vi "MKS_PDR2000_write_read.vi"(0 "PDR2000 COM port":refnum<visa-resource-name>, 2 "Write string":string, 11 "error in (no error)":errorcluster) -> (4 "PDR2000 COM port out":refnum<visa-resource-name>, 13 "Read String":string, 15 "error out":errorcluster)   [LabVIEW 2019]
uses:
  <vilib>/regexp/Match Regular Expression.xnode
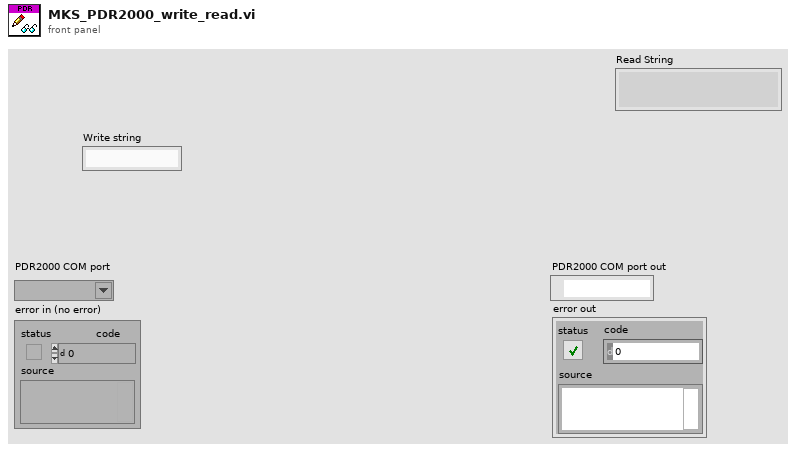
[diagram p1: front panel]
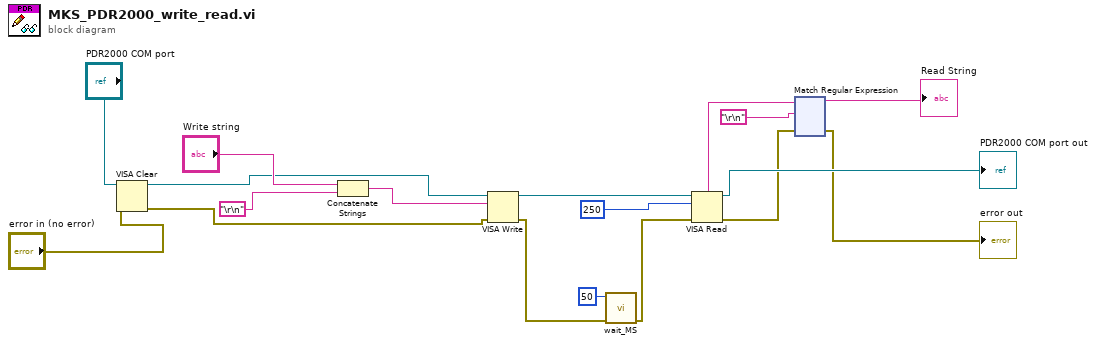
[diagram p0: block diagram]
diagram:
  n1 = VISA Clear(VISA resource name="PDR2000 COM port", error in (no error)="error in (no error)") -> (VISA resource name out=w4:refnum<visa-resource-name>, error out=w3:errorcluster)
  n2 = Concatenate Strings("Write string", "\r\n") -> (w17:string)
  n3 = VISA Write(VISA resource name=w4, write buffer=w17, error in (no error)=w3) -> (VISA resource name out=w14:refnum<visa-resource-name>, error out=w16:errorcluster)  [unwired: 1 out]
  n4 = call "wait_MS.vi"("error in (no error)"=w16, "milliseconds to wait"=u32 50) -> ("error out"=w15:errorcluster)  [unwired: 9 in]
  n5 = VISA Read(VISA resource name=w14, byte count=u32 250, error in (no error)=w15) -> (VISA resource name out=→"PDR2000 COM port out":refnum<visa-resource-name>, read buffer=w10:string, error out=w8:errorcluster)  [unwired: 1 out]
  n6 = xnode "Match Regular Expression"("input string"=w10, "regular expression"="\r\n", "error in"=w8) -> ("before match"=→"Read String":string, "error out"=→"error out":errorcluster)  [unwired: 3 in, 3 out]
